vi "validate line configuration.vi"(7 "modbus":refnum<class "Modbus Module configuration.lvclass">, 11 "line in":T1) -> (1 "valid?":bool, 2 "issues":string, 3 "line out":T1)   [LabVIEW 2013, in "Modbus Module editor node.lvclass"]
doc: "Platypus Framework 1.0.1.65\nNI Systems Engineering - National Instruments"
uses:
  Modbus Module editor node.lvclass
  table line.ctl
  module/module channel/Modbus Module Channel.lvclass
  module/configuration/Modbus Module configuration.lvclass
  module/configuration/Modbus Module configuration.lvclass/Modbus Module configuration.ctl
  <vilib>/NI/Tag Bus/tag/tag descriptor.lvclass/tag descriptor.ctl
  module/module channel/Modbus Module Channel.lvclass/Modbus Module Channel.ctl
  <vilib>/NI/Tag Bus/tag/Data Type.ctl
  <vilib>/NI/Tag Bus/tag/read tag name.vi
  module/module channel/Read modbus type.vi
  module/module channel/Read starting address.vi
  <vilib>/NI/Tag Bus/tag/read data type.vi
  module/module channel/Read subindex (bool).vi
  <vilib>/NI/Tag Bus/tag/tag descriptor.lvclass
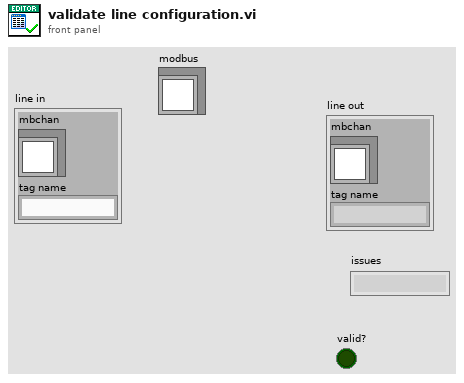
[diagram p1: front panel]
types:
  T1 = typedef "Modbus Module editor node.lvclass/table line.ctl" = cluster{"mbchan":refnum<class "Modbus Module Channel.lvclass">, "tag name":string}
  T2 = typedef "tag bus.lvlib/tag descriptor.lvclass/Data Type.ctl" = enum16{"Double", "Single", "I64", "I32", "I16", "I8", "U64", "U32", "U16", "U8", "Boolean", "String", "Array of Double", "Array of Single", "Array of I64", "Array of I32", "Array of I16", "Array of I8", "Array of U64", "Array of U32", "Array of U16", "Array of U8", "Array of Boolean", "Array of String"}
  T3 = typedef "Modbus Module Channel.lvclass/data bank type.ctl" = enum16{"coils", "discrete inputs", "input registers", "holding registers"}
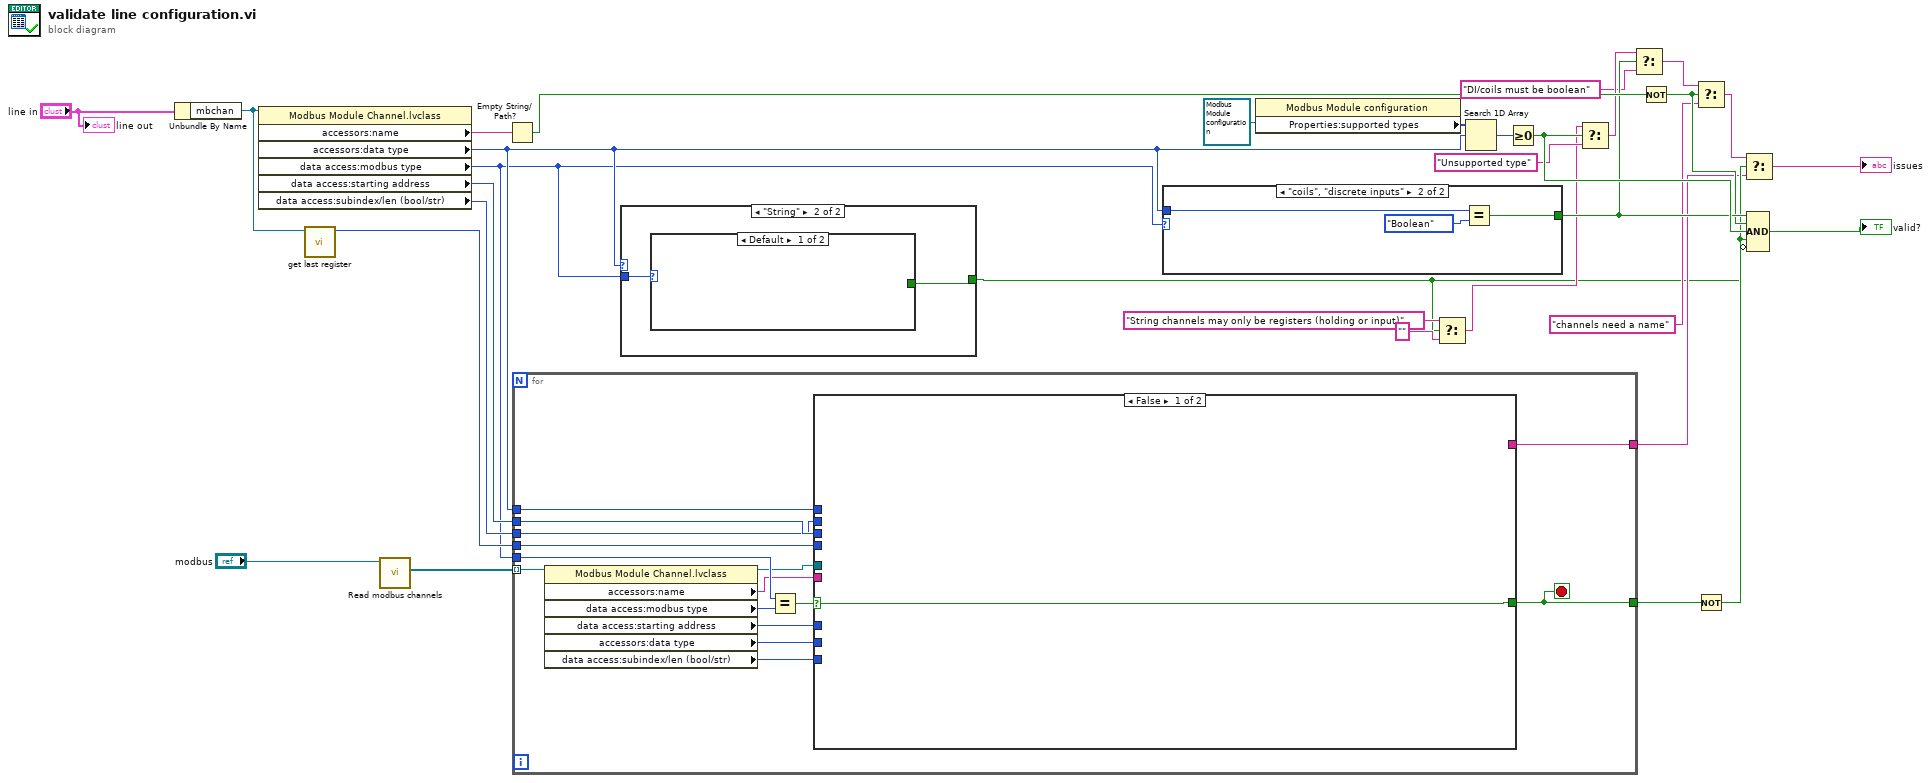
[diagram p0: block diagram]
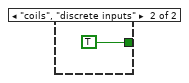
[diagram p3: hidden frame]
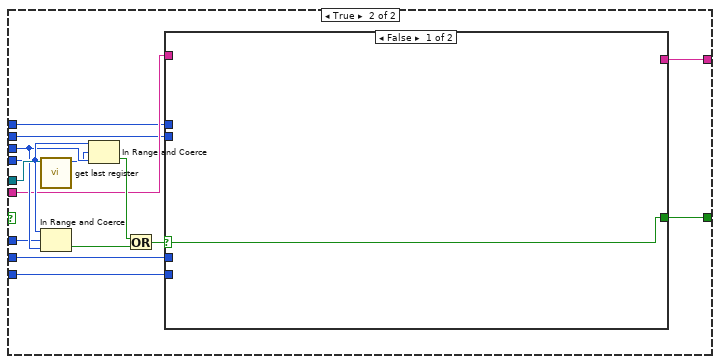
[diagram p4: hidden frame]
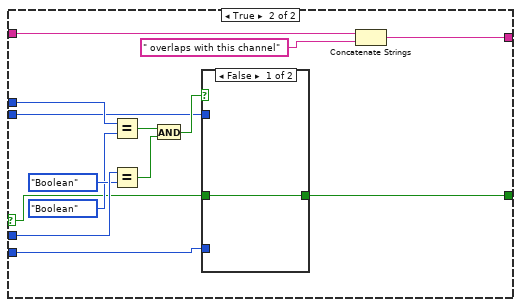
[diagram p5: hidden frame]
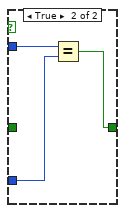
[diagram p6: hidden frame]
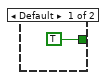
[diagram p7: hidden frame]
diagram:
  n1 = Unbundle By Name("line in") -> ("mbchan"=w17:refnum<class "Modbus Module Channel.lvclass">)
  n2 = property class="Modbus Module Channel.lvclass"(reference=w17) -> ("accessors:name"=w31:string, "accessors:data type"=w6:T2, "data access:modbus type"=w5:T3, "data access:starting address"=w10:u16, "data access:subindex/len (bool/str)"=w7:i32)  [unwired: 1 in, 2 out]
  n3 = call "get last register.vi"("Modbus Module Channel in"=w17) -> ("last element"=w9:i32)  [unwired: 10 in]
  n4 = call "Read modbus channels.vi"("Modbus Slave configuration in"="modbus") -> ("modbus channels"=w16:refnum<class "Modbus Module Channel.lvclass">[])  [unwired: 8 in, 2 out]
  n5 = Empty String/Path?(string/path=w31) -> (empty?=w30:bool)
  n6 = for {
    tunnel: w16 -> [w47] mode=indexing
    tunnel: w5 -> [w45]
    tunnel: [w43] -> w11
    tunnel: w10 -> [w41]
    tunnel: w9 -> [w40]
    tunnel: [w38] -> w8
    tunnel: w6 -> [w35]
    tunnel: w7 -> [w33]
    stop <- w43 stop-if-true
    n7 = property class="Modbus Module Channel.lvclass"(reference=w47) -> (reference out=w42:refnum<class "Modbus Module Channel.lvclass">, "accessors:name"=w37:string, "data access:modbus type"=w46:T3, "data access:starting address"=w39:u16, "accessors:data type"=w36:T2, "data access:subindex/len (bool/str)"=w34:i32)  [unwired: 1 in, 1 out]
    n8 = Equal?(x=w45, y=w46) -> (x = y?=w44:bool)
    n9 = case shown="False" w44 {
      selector: w44 -> [w48 _]
      tunnel: [w48 w54] -> w43
      tunnel: w42 -> [_ w63]
      tunnel: w41 -> [_ w61]
      tunnel: w40 -> [_ w62]
      tunnel: w39 -> [_ w59]
      tunnel: [_ w55] -> w38
      tunnel: w37 -> [_ w53]
      tunnel: w36 -> [_ w52]
      tunnel: w35 -> [_ w51]
      tunnel: w34 -> [_ w50]
      tunnel: w33 -> [_ w49]
      frame False {
      }
      frame True {
        n10 = call "get last register.vi"("Modbus Module Channel in"=w63) -> ("last element"=w60:i32)  [unwired: 10 in]
        n11 = In Range and Coerce(upper limit=w62, x=w59, lower limit=w61) -> (In Range?=w57:bool)  [unwired: 1 out]
        n12 = In Range and Coerce(upper limit=w62, x=w60, lower limit=w61) -> (In Range?=w58:bool)  [unwired: 1 out]
        n13 = Or(x=w58, y=w57) -> (x .or. y?=w56:bool)
        n14 = case shown="False" w56 {
          selector: w56 -> [w64 w70]
          tunnel: [_ w66] -> w55
          tunnel: [w64 w71] -> w54
          tunnel: w53 -> [_ w65]
          tunnel: w52 -> [_ w78]
          tunnel: w51 -> [_ w75]
          tunnel: w50 -> [_ w69]
          tunnel: w49 -> [_ w68]
          frame False {
          }
          frame True {
            n15 = Equal?(x=w75, y=Data_Type."Boolean") -> (x = y?=w74:bool)
            n16 = Equal?(x=w78, y=Data_Type."Boolean") -> (x = y?=w73:bool)
            n17 = And(x=w74, y=w73) -> (x .and. y?=w72:bool)
            n18 = case shown="False" w72 {
              tunnel: [w79 w80] -> w71
              tunnel: w70 -> [w79 _]
              tunnel: w69 -> [_ w81]
              tunnel: w68 -> [_ w82]
              frame False {
              }
              frame True {
                n19 = Equal?(x=w82, y=w81) -> (x = y?=w80:bool)
              }
            }
            n20 = Concatenate Strings(w65, " overlaps with this channel" ("string")) -> (w66:string)
          }
        }
      }
    }
  }
  n21 = case shown="\"String\"" w6 {
    tunnel: w5 -> [_ w84]
    tunnel: [_ w83] -> w1
    frame "Double", Default {
    }
    frame "String" {
      n22 = case shown="Default" w84 {
        tunnel: [_ TRUE] -> w83
        frame Default {
        }
        frame "coils", "discrete inputs" {
        }
      }
    }
  }
  n23 = case shown="\"coils\", \"discrete inputs\"" w5 {
    tunnel: [TRUE w89] -> w22
    tunnel: w6 -> [_ w88]
    frame Default {
    }
    frame "coils", "discrete inputs" {
      n24 = Equal?(x=w88, y=Data_Type."Boolean") -> (x = y?=w89:bool)
    }
  }
  n25 = property class="Modbus Module configuration"(reference=refnum<class "Modbus Module configuration.lvclass"> refnum ("tag bus configurable plugin module configuration")) -> ("Properties:supported types"=w28:T2[])  [unwired: 1 in, 2 out]
  n26 = Select(t="String channels may only be registers (holding or input)", s=w1, f="") -> (s? t:f=w3:string)
  n27 = Search 1D Array(1D array=w28, element=w6) -> (index of element=w26:i32)  [unwired: 1 in]
  n28 = Greater Or Equal To 0?(x=w26) -> (x >= 0?=w25:bool)
  n29 = Select(t=w3, s=w25, f="Unsupported type") -> (s? t:f=w23:string)
  n30 = Select(t=w23, s=w22, f="DI/coils must be boolean") -> (s? t:f=w20:string)
  n31 = Not(x=w30) -> (.not. x?=w19:bool)
  n32 = Select(t=w20, s=w19, f="channels need a name") -> (s? t:f=w14:string)
  n33 = Not(x=w11) -> (.not. x?=w12:bool)
  n34 = Select(t=w14, s=w12, f=w8) -> (s? t:f=→"issues":string)
  n35 = Compound Arithmetic op=AND(w22, w19, w25, w12, invert w1) -> (→"valid?":bool)
  "line out" <- "line in"
